vi "ritter reset.vi"(8 "error in (no error)":errorcluster, 11 "VISA in":refnum<visa-resource-name>) -> (0 "error out":errorcluster, 3 "VISA out":refnum<visa-resource-name>)   [LabVIEW 2023]
doc: "This vi returns the current flow through the Ritter gasmeter."
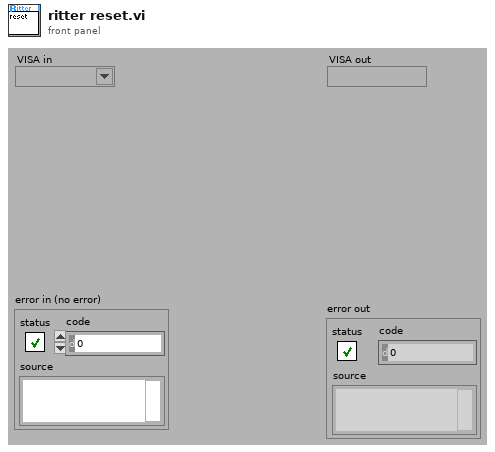
[diagram p1: front panel]
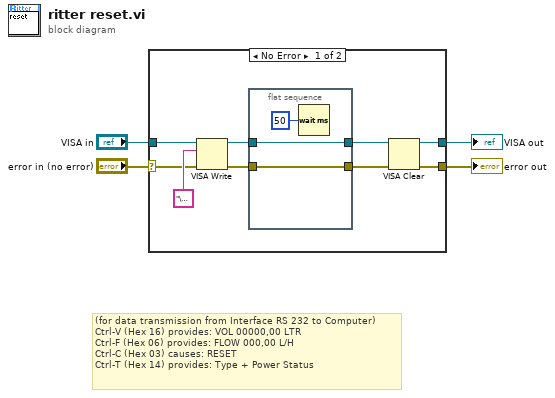
[diagram p0: block diagram]
diagram:
  # "(for data transmission from Interface RS 232 to Computer)\nCtrl-V (Hex 16) provides: VOL 00000,00 LTR\nCtrl-F (Hex 06) provides: FLOW 000,00 L/H\nCtrl-C (Hex 03) causes: RESET\nCtrl-T (Hex 14) provides: Type + Power Status"
  n1 = case shown="No Error" "error in (no error)" {
    selector: "error in (no error)" -> [w5 w17]
    tunnel: "VISA in" -> [w10 w18]
    tunnel: [w7 w17] -> w3
    tunnel: [w6 w18] -> w2
    frame No Error {
      n2 = VISA Write(VISA resource name=w10, write buffer="\u0003" ("string"), error in (no error)=w5) -> (VISA resource name out=w11:refnum<visa-resource-name>, error out=w12:errorcluster)  [unwired: 1 out]
      n3 = flat-sequence {
        tunnel: w12 -> [w16]
        tunnel: [w16] -> w8
        tunnel: w11 -> [w15]
        tunnel: [w15] -> w9
        frame #0 {
          n4 = Wait (ms)(milliseconds to wait=u32 50) -> ()  [unwired: 1 out]
        }
      }
      n5 = VISA Clear(VISA resource name=w9, error in (no error)=w8) -> (VISA resource name out=w6:refnum<visa-resource-name>, error out=w7:errorcluster)
    }
    frame Error {
    }
  }
  "error out" <- w3
  "VISA out" <- w2
